vi "Save Image as any type.vi"(8 "error in":errorcluster, 9 "File Type":T2, 10 "File Path":path, 11 "Image":T1) -> (0 "error out":errorcluster, 3 "Image Out":T1)   [LabVIEW 2015, in "Camera SubVIs.lvlib"]
uses:
  Camera SubVIs.lvlib
  <vilib>/vision/Image Controls.llb/IMAQ Image.ctl
  Image File Type.ctl
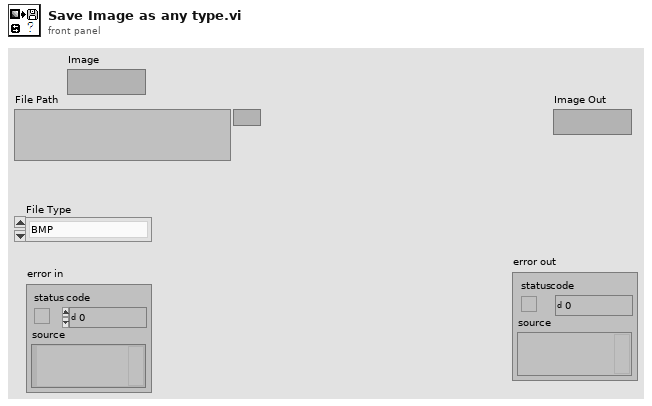
[diagram p1: front panel]
types:
  T1 = typedef "IMAQ Image.ctl" = refnum<image>
  T2 = typedef "Camera SubVIs.lvlib/Image File Type.ctl" = enum16{"BMP", "JPEG", "JPEG 2000", "PNG", "PNG with Vision Info", "TIFF"}
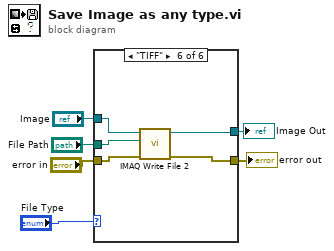
[diagram p0: block diagram]
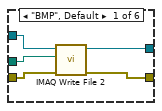
[diagram p2: hidden frame]
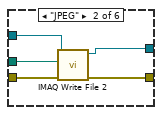
[diagram p3: hidden frame]
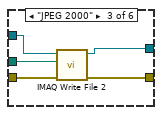
[diagram p4: hidden frame]
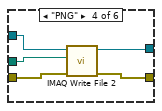
[diagram p5: hidden frame]
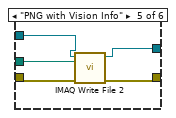
[diagram p6: hidden frame]
diagram:
  n1 = case shown="\"TIFF\"" "File Type" {
    tunnel: "File Path" -> [w10 w16 w19 w24 w29 w34]
    tunnel: "Image" -> [w11 w15 w21 w26 w31 w33]
    tunnel: [w8 w14 w17 w22 w27 w35] -> w4
    tunnel: "error in" -> [w9 w13 w18 w23 w28 w36]
    tunnel: [w7 w12 w20 w25 w30 w32] -> w1
    frame "BMP", Default {
      n2 = call-poly "IMAQ Write File 2"("error in (no error)"=w9, "File Path"=w10, "Image"=w11) -> ("error out"=w8:errorcluster, "Image Out (duplicate)"=w7:T1)  [unwired: 7 in]
    }
    frame "JPEG" {
      n3 = call-poly "IMAQ Write File 2"("error in (no error)"=w13, "File Path"=w16, "Image"=w15) -> ("error out"=w14:errorcluster, "Image Out (duplicate)"=w12:T1)  [unwired: 7 in]
    }
    frame "JPEG 2000" {
      n4 = call-poly "IMAQ Write File 2"("error in (no error)"=w18, "File Path"=w19, "Image"=w21) -> ("error out"=w17:errorcluster, "Image Out (duplicate)"=w20:T1)  [unwired: 7 in]
    }
    frame "PNG" {
      n5 = call-poly "IMAQ Write File 2"("error in (no error)"=w23, "File Path"=w24, "Image"=w26) -> ("error out"=w22:errorcluster, "Image Out (duplicate)"=w25:T1)  [unwired: 7 in]
    }
    frame "PNG with Vision Info" {
      n6 = call-poly "IMAQ Write File 2"("error in (no error)"=w28, "File Path"=w29, "Image"=w31) -> ("error out"=w27:errorcluster, "Image Out (duplicate)"=w30:T1)  [unwired: 7 in]
    }
    frame "TIFF" {
      n7 = call-poly "IMAQ Write File 2"("error in (no error)"=w36, "File Path"=w34, "Image"=w33) -> ("error out"=w35:errorcluster, "Image Out (duplicate)"=w32:T1)  [unwired: 7 in]
    }
  }
  "error out" <- w4
  "Image Out" <- w1
